vi "ICR_Run_Sequence.vi"(8 "error in (no error)":errorcluster caption="error in", 11 "QMH ICR Cluster":T2) -> (0 "error out":errorcluster, 3 "QMH ICR Cluster":T2)   [LabVIEW 2024]
doc: "This VI starts the hardware boards in asynchronous mode: the OS is not waiting for the board response.\nAll boards are waiting for the triggers of the sequencer HSDIO.\nAn event \"Disk written done\" is generated when the current accumulation is finished."
uses:
  controls/QMH_ICR_Cluster.ctl
  controls/HARDWARE_Resources.ctl
  controls/PROCESSING_Inputs.ctl
  controls/LOOPS_Inputs.ctl
  controls/OPO_Inputs.ctl
panel:
  in  "HARDWARE Resources":T1={"AO6711 Physical Channels"="Analog/ao0:3", "AO6711 Task Name"="", "AWG5421 Resource Name"="Waveform", "DIGIT 5122 Resource Name"="Digitizer", "HSDIO Resource Name"="Sequencer"}
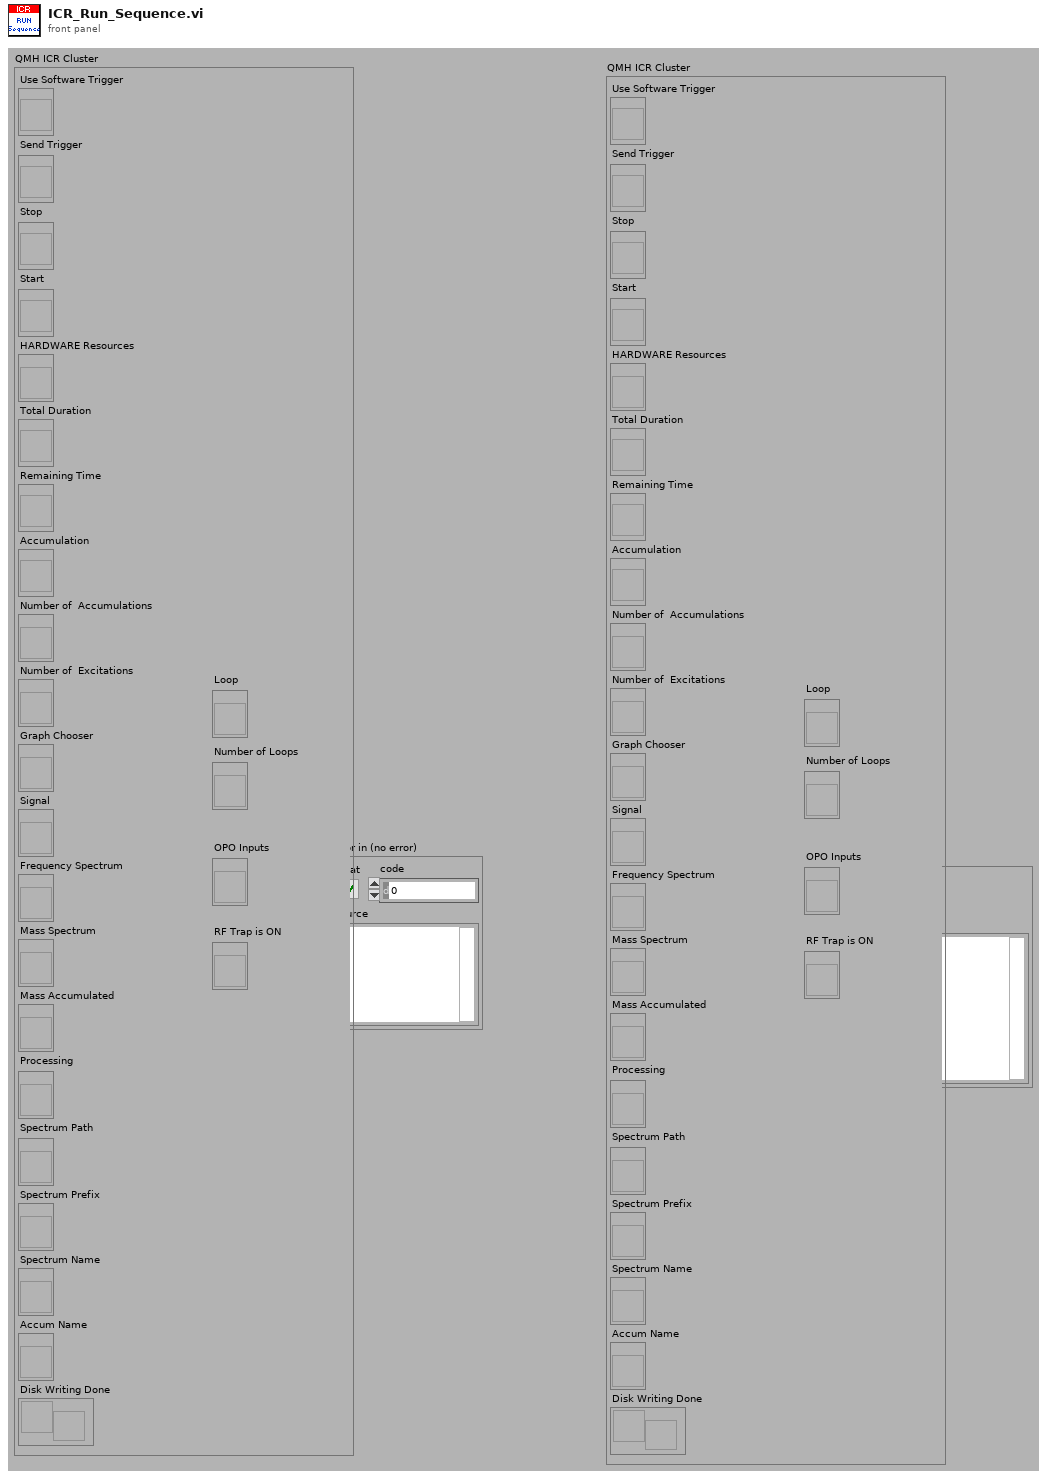
[diagram p1: front panel]
types:
  T1 = typedef "HARDWARE_Resources.ctl" = cluster{"AO6711 Physical Channels":tag, "AO6711 Task Name":refnum<k21>, "AWG5421 Resource Name":refnum<k15>, "DIGIT 5122 Resource Name":refnum<k15>, "HSDIO Resource Name":refnum<k15>}
  T2 = typedef "QMH_ICR_Cluster.ctl" = cluster{"Use Software Trigger":refnum<vi>, "Send Trigger":refnum<vi>, "Stop":refnum<vi>, "Start":refnum<vi>, "HARDWARE Resources":refnum<vi>, "Total Duration":refnum<vi>, "Remaining Time":refnum<vi>, "Accumulation":refnum<vi>, "Number of  Accumulations":refnum<vi>, "Number of  Excitations":refnum<vi>, "Graph Chooser":refnum<vi>, "Signal":refnum<vi>, "Frequency Spectrum":refnum<vi>, "Mass Spectrum":refnum<vi>, "Mass Accumulated":refnum<vi>, "Processing":refnum<vi>, "Spectrum Path":refnum<vi>, "Spectrum Prefix":refnum<vi>, "Spectrum Name":refnum<vi>, "Accum Name":refnum<vi>, "Disk Writing Done":refnum<notifier>, "Loop":refnum<vi>, "Number of Loops":refnum<vi>, "OPO Inputs":refnum<vi>, "RF Trap is ON":refnum<vi>}
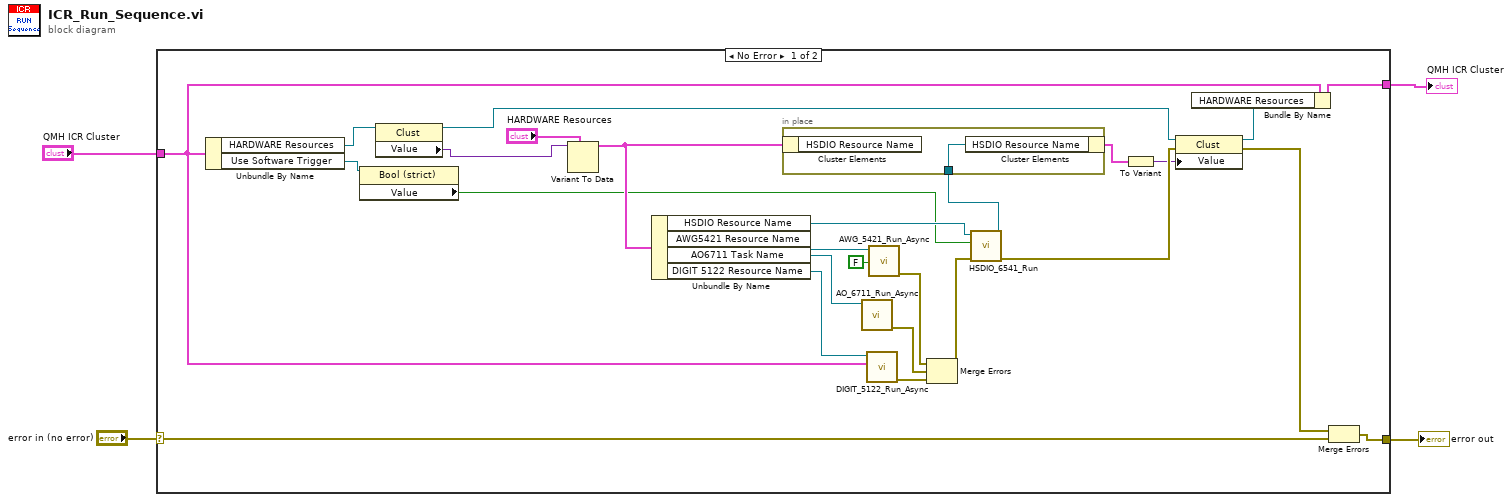
[diagram p0: block diagram]
diagram:
  n1 = case shown="No Error" "error in (no error)" {
    selector: "error in (no error)" -> [w28 w33]
    tunnel: [w27 w33] -> w4
    tunnel: "QMH ICR Cluster" -> [w8 w32]
    tunnel: [w6 w32] -> w1
    frame No Error {
      n2 = Unbundle By Name(w8) -> ("HARDWARE Resources"=w17:refnum<vi>, "Use Software Trigger"=w16:refnum<vi>)
      n3 = property class="Bool (strict)"(reference=w16) -> ("Value"=w9:bool)  [unwired: 1 in, 2 out]
      n4 = property class="Clust"(reference=w17) -> (reference out=w18:refnum<vi>, "Value"=w22:variant)  [unwired: 1 in, 1 out]
      n5 = Variant To Data(type="HARDWARE Resources", Variant=w22) -> (data=w20:T1)  [unwired: 1 in, 1 out]
      n6 = Unbundle By Name(w20) -> ("HSDIO Resource Name"=w30:refnum<k15>, "AWG5421 Resource Name"=w26:refnum<k15>, "AO6711 Task Name"=w12:refnum<k21>, "DIGIT 5122 Resource Name"=w13:refnum<k15>)
      n7 = call "AO_6711_Run_Async.vi"("Instrument handle in"=w12) -> ("error out"=w10:errorcluster)  [unwired: 10 in]
      n8 = call "DIGIT_5122_Run_Async.vi"("QMH ICR Cluster"=w8, "instrument handle in"=w13) -> ("error out"=w11:errorcluster)  [unwired: 9 in]
      n9 = call "AWG_5421_Run_Async.vi"("Use Software trigger"=FALSE, "AWG5421 Resource Name"=w26) -> ("error out"=w23:errorcluster)  [unwired: 9 in]
      n10 = Merge Errors(w23, w10, w11) -> (w24:errorcluster)
      n11 = call "HSDIO_6541_Run.vi"("error  in"=w24, "Use Software trigger"=w9, "instrument handle in"=w30) -> ("error out"=w15:errorcluster, "instrument handle out"=w29:refnum<k15>)  [unwired: 7 in]
      n12 = in-place {
        in-place-border: w29 -> [w31]
        n13 = in-place-cluster #1(w20) -> ()  [unwired: 1 out]
        n14 = in-place-cluster #1("HSDIO Resource Name"=w31) -> (w19:T1)
      }
      n15 = To Variant(anything=w19) -> (Variant=w7:variant)
      n16 = property class="Clust"(reference=w18, error in=w15, "Value"=w7) -> (reference out=w5:refnum<vi>, error out=w14:errorcluster)
      n17 = Bundle By Name(cluster=w8, "HARDWARE Resources"=w5) -> (w6:T2)
      n18 = Merge Errors(w14, w28) -> (w27:errorcluster)
    }
    frame Error {
    }
  }
  "error out" <- w4
  "QMH ICR Cluster" <- w1
